vi "Compile HW Channel Data.vi"(8 "error in (no error)":errorcluster, 11 "Desired Values Refs":T4[](array[typedef]) format="%.0x") -> (0 "error out":errorcluster, 2 "Compiled HW Channels":T1[](array[typedef]))   [LabVIEW 2017, in "NI 272x Resistive Simulation Custom Device Configuration.lvlib"]
uses:
  NI 272x Resistive Simulation Custom Device Configuration.lvlib
  <vilib>/NI Veristand/Custom Device API/Custom Device Item Ref.ctl
  Controls/Compiled HW Channel.ctl
  Controls/Channel Mode.ctl
  <instrlib>/ni272xReferenceVIs/ni272xReferenceVIs.llb/ni272x Callendar-Van Dusen RTD Parameters.ctl
  Globals/Names.vi
  <vilib>/NI Veristand/Custom Device API/Get Item Property (U16).vi
  NI 272x Resistive Simulation Custom Device Shared.lvlib
  <vilib>/NI VeriStand/Custom Device API/Custom Device API.lvlib
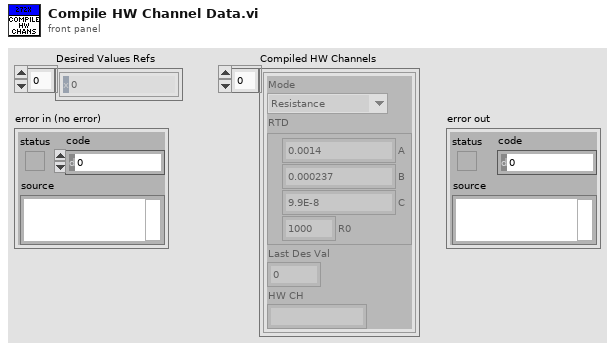
[diagram p1: front panel]
types:
  T1 = typedef "NI 272x Resistive Simulation Custom Device Shared.lvlib/Compiled HW Channel.ctl" = cluster{"Mode":T2, "RTD":T3, "Last Des Val":dbl, "HW CH":string}
  T2 = typedef "NI 272x Resistive Simulation Custom Device Shared.lvlib/Channel Mode.ctl" = enum16{"Resistance", "RTD Temperature"}
  T3 = typedef "ni272x Callendar-Van Dusen RTD Parameters.ctl" = cluster{"A":dbl, "B":dbl, "C":dbl, "R0":dbl}
  T4 = typedef "Custom Device API.lvlib/Custom Device Item Ref.ctl" = u64
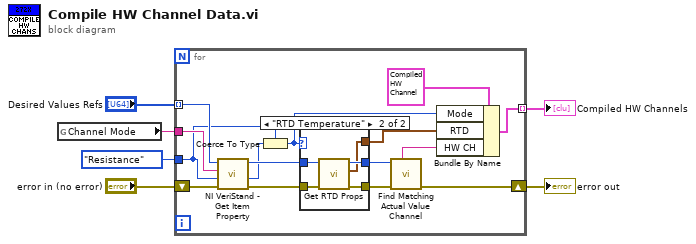
[diagram p0: block diagram]
diagram:
  n1 = global read "Names.vi" "Channel Mode"() -> (w5:string)
  n2 = for {
    tunnel: "Desired Values Refs" -> [w18] mode=indexing
    tunnel: w5 -> [w17]
    tunnel: Channel_Mode."Resistance" ("Mode") -> [w12]
    shift-right: [w8] -> w2
    shift-left: "error in (no error)" -> [w21]
    tunnel: [w9] -> w1 mode=indexing
    n3 = call-poly <vilib>:"NI VeriStand - Get Item Property.vi"("error in (no error)"=w21, "Default Value"=w12, "Property Name"=w17, "Item Ref in"=w18) -> ("error out"=w19:errorcluster, "Value"=w13:u16, "Item Ref out"=w15:T4)  [unwired: 4 in, 1 out]
    n4 = Coerce To Type(0:w13, 1:w12) -> (2:w11:T2)
    n5 = case shown="\"RTD Temperature\"" w11 {
      tunnel: w19 -> [w23 w28]
      tunnel: [w23 w27] -> w16
      tunnel: w15 -> [w22 w26]
      tunnel: [w22 w25] -> w14
      tunnel: [_ w24] -> w10
      frame "Resistance" {
      }
      frame "RTD Temperature" {
        n6 = call "Get RTD Props.vi"("error in (no error)"=w28, "Item Ref in"=w26) -> ("error out"=w27:errorcluster, "temp param"=w24:T3, "Item Ref out"=w25:T4)  [unwired: 7 in]
      }
    }
    n7 = call "Find Matching Actual Value Channel.vi"("error in (no error)"=w16, "Desired item ref in"=w14) -> ("error out"=w8:errorcluster, "CH#"=w7:string)  [unwired: 4 in, 4 out]
    n8 = Bundle By Name(cluster=T1 {"Mode"=enum."Resistance", "RTD"={"A"=0.0, "B"=0.0, "C"=0.0, "R0"=0.0}, "Last Des Val"=0.0, "HW CH"=""} ("HW Chn"), "Mode"=w11, "RTD"=w10, "HW CH"=w7) -> (w9:T1)
  }
  "error out" <- w2
  "Compiled HW Channels" <- w1
